vi "BarChart.vi"(11 "Array":u8[](array[numeric])) -> (1 "X frame matrix":u8[](array[numeric]), 3 "XY Graph":cluster{i32[], i32[]}(graph))   [LabVIEW 2014]
panel:
  out "cy":i32
  out "y1":i32
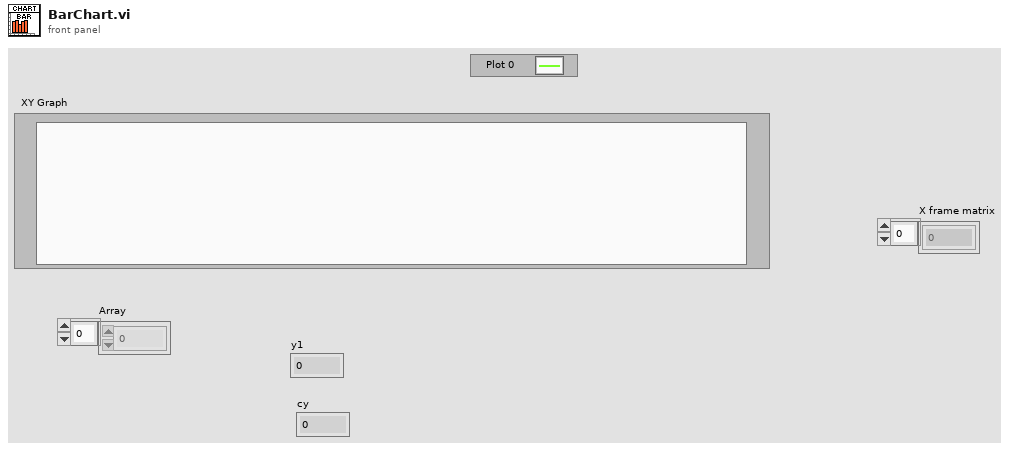
[diagram p1: front panel]
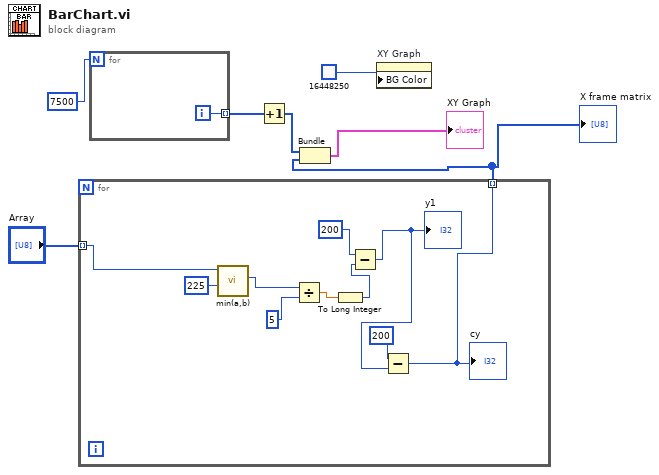
[diagram p0: block diagram]
diagram:
  n1 = for {
    tunnel: "Array" -> [w17] mode=indexing
    tunnel: [w8] -> w1 mode=indexing
    n2 = call "min(a,b).vi"("b"=u8 225, "a"=w17) -> ("Out"=w15:u8)  [unwired: 9 in]
    n3 = Divide(x=w15, y=u8 5) -> (x/y=w12:dbl)
    n4 = To Long Integer(number=w12) -> (32bit integer=w11:i32)
    n5 = Subtract(x=200, y=w11) -> (x-y=w10:i32)
    "y1" <- w10
    n6 = Subtract(x=200, y=w10) -> (x-y=w8:i32)
    "cy" <- w8
  }
  "X frame matrix" <- w1
  n7 = for {
    N: 7500 -> [_]
    tunnel: [w18] -> w5 mode=indexing
    i -> [w18]
  }
  n8 = Increment(x=w5) -> (x+1=w2:i32[])
  n9 = Bundle(w2, w1) -> (→"XY Graph":cluster{i32[], i32[]})  [unwired: 1 in]
  n10 = property on="XY Graph" class="XYGraph (strict)"("BG Color"=u32 16448250) -> ()  [unwired: 2 in, 2 out]
